vi "Main Loop.vi"(8 "error in (no error)":errorcluster, 10 "Chart Notifier":refnum<notifier>, 11 "Message Queues":T1) -> (0 "error out":errorcluster)   [LabVIEW 2018, in "Feed Module.lvlib" / "Feed Module Engine.lvlib"]
uses:
  Feed Module Engine.lvlib
  Feed Module/Controls/Feed Message Queues.ctl
  support/Message Queue/Message Cluster.ctl
  State Cluster.ctl
  State Enum.ctl
  Feed Module/Controls/Feed Module Settings Cluster.ctl
  Ismatec ISM 831C/Controls/Ismatech ISM831C Settings Cluster.ctl
  Masterflex 7550-30/Controls/Settings Cluster.ctl
  Mettler Toledo/Controls/Settings Cluster.ctl
  Bronkhorst M13 Flow Meter/Settings Cluster.ctl
  PID 2 Parameters Cluster.ctl
  PID Input Enum.ctl
  PID 2 Output Enum.ctl
  Tacmina QI/Tacmina QI DAQ Setting.ctl
  KNF Pump/Settings Cluster plus SIMDOS.ctl
  ASIA Pump/Pump Settings.ctl
  VICI M50 Party Mode/Settings Cluster.ctl
  FLOM Pump/Settings Cluster.ctl
  SSI PR Class/SSI PR or LD Settings Cluster.ctl
  Masterflex 75211/Masterflex 75211 DAQ Setting.ctl
  SSI PR Class/SSI P40 Settings Cluster.ctl
  Ismatec 78001/Ismatec 4083.ctl
  Bronkhorst M14 Flow Meter/Settings Cluster.ctl
  PID 1 Parameters Cluster.ctl
  Feed Module/Controls/Feed Module Display.ctl
  Config Module/Controls/OP Window Display.ctl
  <vilib>/Platform/TimedLoop/XDataNode/timing_clust.ctl
  <vilib>/Platform/TimedLoop/XDataNode/nitl_modes.ctl
  <vilib>/Platform/TimedLoop/XDataNode/wakeup.ctl
  Tag VIs/Tag FGV Operation Enum.ctl
  support/Message Queue/Enqueue Message (Single).vi
  <vilib>/Platform/TimedLoop/XDataNode/XDataNode.xnode
  support/Message Queue/Message Queue.lvlib
  <vilib>/Platform/TimedLoop/XDataNode/XDNodeRunTimeDep.lvlib
  Feed Module/Feed Module.lvlib
  Ismatec ISM 831C/Ismatec ISM 831C.lvlib
  Masterflex 7550-30/Masterflex 7550-30.lvlib
  Bronkhorst M13 Flow Meter/Bronkhorst M13 Flow Meter.lvlib
  Mettler Toledo/Mettler Toledo.lvlib
  Tacmina QI/Tacmina QI.lvlib
  Shared Variables/Dynamic Shared Variables.lvlib
  KNF Pump/KNF SIMDOS.lvlib
  ASIA Pump.lvlib
  VICI M50 Party Mode/VICI M6 M50 Party Mode.lvlib
  FLOM Pump/FLOM Pump.lvlib
  SSI PR Class/SSI PR or LD Pump.lvlib
  support/Support Library.lvlib
  Masterflex 75211/Masterflex 75211.lvlib
  SSI PR Class/SSI P40 Pump.lvlib
  Ismatec 78001/Ismatec 4308.lvlib
  Bronkhorst M14 Flow Meter/Bronkhorst M14 Flow Meter.lvlib
panel:
  out "Period (s)":dbl format="%_4g"
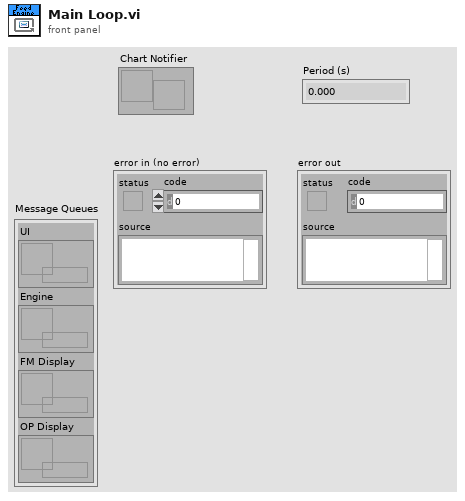
[diagram p1: front panel]
types:
  T1 = typedef "Feed Module.lvlib/Feed Message Queues.ctl" = cluster{"UI":refnum<queue>, "Engine":refnum<queue>, "FM Display":refnum<queue>, "OP Display":refnum<queue>}
  T2 = typedef "XDNodeRunTimeDep.lvlib/timing_clust.ctl" = cluster{"Expected End [f-1]":u64, "Actual End [f-1]":u64, "Finished Late? [f-1]":bool, "Expected End [i-1]":u64, "Actual End [i-1]":u64, "Finished Late? [i-1]":bool, "Expected Start [i]":u64, "Actual Start [i]":u64, "Expected Start [f]":u64, "Actual Start [f]":u64, "Source Name":string, "Structure Name":string, "Period":i64, "Deadline":i64, "Offset":i64, "Start":i64, "Priority":i32, "Timeout":i32, "Mode":T3, "Wakeup Reason":T4, "Error":errorcluster, "Source Type":string, "Secondary Source Type":string, "Global End Time":u64, "Global Start Time":u64, "Frame Duration":u64, "Iteration Duration":u64, "Assigned CPU":i32, "I/O Scan Engine Mode":u32}
  T3 = typedef "XDNodeRunTimeDep.lvlib/nitl_modes.ctl" = enum32{"No Change", "Process missed periods, maintain original phase", "Discard missed periods, maintain original phase", "Process missed periods, ignore original phase", "Discard missed periods, ignore original phase"}
  T4 = typedef "XDNodeRunTimeDep.lvlib/wakeup.ctl" = enum32{"Normal", "Aborted", "Asynchronous wakeup", "Timing source error", "Timed loop error", "Timeout"}
  T5 = cluster{"enable? (F)":bool, "name":string, "alarm on":bool, "priority":u32, "ack type":enum16{"Auto", "User", "None", "Each Occurrence"}, "area":string, "description":string, "log? (T)":bool}
  T6 = typedef "Tag FGV Operation Enum.ctl" = enum16{"Init", "Set Notification Queue", "Create Tag", "Commit", "Write Tag (Numeric)", "Write Tag (Boolean)", "Read All Tags", "Read One Tag", "Delete Tag Category", "Set Alarm Parameters (Numeric)", "Set Alarm Parameters (Boolean)", "Enable All Alarms", "Disable All Alarms", "Delete All Tags", "Read Alarms", "Ack Alarm", "Read Alarm Parameters (Numeric)", "Read Alarm Parameters (Boolean)"}
  T7 = enum32{"u32BitField", "bool", "double", "string", "int8", "uint8", "int16", "uint16", "int32", "uint32", "int64", "uint64", "single", "double waveform", "int16 waveform", "array of boolean", "array of int8", "array of uint8", "array of int16", "array of uint16", "array of int32", "array of uint32", "array of int64", "array of uint64", "array of single", "array of double", "array of double waveform", "array of int16 waveform", "array of string", "variant", "timestamp", "fixed point", "custom"}
  T8 = typedef "Feed Module.lvlib/Feed Module Engine.lvlib/State Enum.ctl" = enum16{"Measuring", "Idle", "Paused"}
  T9 = typedef "Feed Module.lvlib/OP Window Display.ctl" = cluster{"Flow":dbl, "Manual":dbl, "Pump Status":u16, "Smoothed Array":dbl[]}
  T10 = typedef "Feed Module.lvlib/Feed Module Display.ctl" = cluster{"Flow":dbl, "Density":dbl, "FL Temp":dbl, "Scale Value":dbl, "Pump On?":enum16{"Off", "On", "Not Initialized"}, "Cycle Period":dbl, "Input Device":T11, "Output":T12, "Pump's Pressure":dbl, "Pump's Flow ":dbl}
  T11 = typedef "PID Input Enum.ctl" = enum16{"Default", "Bronkhorst M13", "Bronkhorst M14", "Scale Rate of Change"}
  T12 = typedef "PID 2 Output Enum.ctl" = enum16{"Default", "Ismatec ISM 4308", "Ismatec ISM 831C", "Masterflex 7550-30", "VICI", "Tacmina QI", "KNF SIMDOS", "ASIA Type C", "FLOM UI-22-11", "SSI PR/LD", "SSI P40", "Masterflex 75211-70"}
  T13 = typedef "Feed Module.lvlib/Feed Module Engine.lvlib/State Cluster.ctl" = cluster{"State":T8, "Start Time":timestamp, "Configuration":T14, "Current Time":timestamp, "PID 1 Parameters":T30, "First Iteration":bool, "Data":cluster{"Flowmeter Output":dbl, "Density":dbl, "FL Temp":dbl, "Scale Output (g)":dbl, "Scale Rate of Change (g/min)":dbl, "PID 1 Output":dbl, "PID 2 Process Variable":dbl, "PID 2 output":dbl, "Pump Flow":dbl, "Pump Pressure":dbl}, "Process Name":string, "Pump On?":enum16{"Off", "On", "Not Initialized"}, "Input Error":bool, "Output Error":bool, "Log Started":bool, "Current Setpoint":dbl}
  T14 = typedef "Feed Module.lvlib/Feed Module Settings Cluster.ctl" = cluster{"Cycle Period":dbl, "Ismatech":T15, "Masterflex":T16, "Mettler":T17, "Bronkhorst M13 Flow Meter":T18, "PID 2 Parameters":T19, "Manual Entry":dbl, "Auto?":bool, "output range":cluster{"output high":dbl, "output low":dbl}, "Tacmina Settings":T20, "KNF SIMDOS Settings":T21, "ASIA Pump C":T22, "VICI Settings":T23, "FLOM Settings":T24, "SSI PR/LD Settings":T25, "Masterflex 75211 Settings":T26, "SSI P40 Settings":T27, "Ismatech 3 Channel Settings":T28, "Bronkhorst M14 Settings":T29}
  T15 = typedef "Ismatec ISM 831C.lvlib/Ismatech ISM831C Settings Cluster.ctl" = cluster{"VISA resource name":refnum<visa-resource-name>, "Simulated?":bool, "Pump Number":dbl, "Reverse?":bool}
  T16 = typedef "Masterflex 7550-30.lvlib/Settings Cluster.ctl" = cluster{"VISA resource name":refnum<visa-resource-name>, "Simulated?":bool, "Pump Number":dbl, "Reverse?":bool}
  T17 = typedef "Mettler Toledo.lvlib/Settings Cluster.ctl" = cluster{"VISA resource name":refnum<visa-resource-name>, "Simulated?":bool}
  T18 = typedef "Bronkhorst M13 Flow Meter.lvlib/Settings Cluster.ctl" = cluster{"VISA resource name":refnum<visa-resource-name>, "Simulated?":bool, "Smoothing Steps":i32}
  T19 = typedef "PID 2 Parameters Cluster.ctl" = cluster{"Input Device":T11, "Output Device":T12, "Setpoint":dbl, "PID gains":cluster{"proportional gain (Kc)":dbl, "integral time (Ti, min)":dbl, "derivative time (Td, min)":dbl}}
  T20 = typedef "Tacmina QI.lvlib/Tacmina QI DAQ Setting.ctl" = cluster{"Analog DAQ Task":refnum<k21>, "Digital DAQ Task":refnum<k21>}
  T21 = typedef "KNF SIMDOS.lvlib/Settings Cluster plus SIMDOS.ctl" = cluster{"VISA resource name":refnum<visa-resource-name>, "Simulated?":bool}
  T22 = typedef "ASIA Pump.lvlib/Pump Settings.ctl" = cluster{"ASIA Pump #":i32, "channel":i32, "Simulated":bool}
  T23 = typedef "VICI M6 M50 Party Mode.lvlib/Settings Cluster.ctl" = cluster{"VISA resource name":refnum<visa-resource-name>, "Simulated?":bool, "Pump Letter":string, "Reverse?":bool}
  T24 = typedef "FLOM Pump.lvlib/Settings Cluster.ctl" = cluster{"VISA resource name":refnum<visa-resource-name>, "Simulated?":bool, "Pump Number":dbl}
  T25 = typedef "SSI PR or LD Pump.lvlib/SSI PR or LD Settings Cluster.ctl" = cluster{"VISA resource name":refnum<visa-resource-name>, "Simulated?":bool}
  T26 = typedef "Masterflex 75211.lvlib/Masterflex 75211 DAQ Setting.ctl" = cluster{"Analog DAQ Task":refnum<k21>, "Digital DAQ Task":refnum<k21>}
  T27 = typedef "SSI P40 Pump.lvlib/SSI P40 Settings Cluster.ctl" = cluster{"VISA resource name":refnum<visa-resource-name>, "Simulated?":bool}
  T28 = typedef "Ismatec 4308.lvlib/Ismatec 4083.ctl" = cluster{"VISA resource name":refnum<visa-resource-name>, "Pump Number":i16, "Channel Number":i16, "Simulated?":bool, "Reverse?":bool}
  T29 = typedef "Bronkhorst M14 Flow Meter.lvlib/Settings Cluster.ctl" = cluster{"VISA resource name":refnum<visa-resource-name>, "Simulated?":bool, "Smoothing Steps":i32}
  T30 = typedef "PID 1 Parameters Cluster.ctl" = cluster{"Setpoint":dbl, "PID gains":cluster{"proportional gain (Kc)":dbl, "integral time (Ti, min)":dbl, "derivative time (Td, min)":dbl}}
  T31 = cluster{"Flowmeter Output":dbl, "Density":dbl, "FL Temp":dbl, "Scale Output (g)":dbl, "Scale Rate of Change (g/min)":dbl, "PID 1 Output":dbl, "PID 2 Process Variable":dbl, "PID 2 output":dbl, "Pump Flow":dbl, "Pump Pressure":dbl}
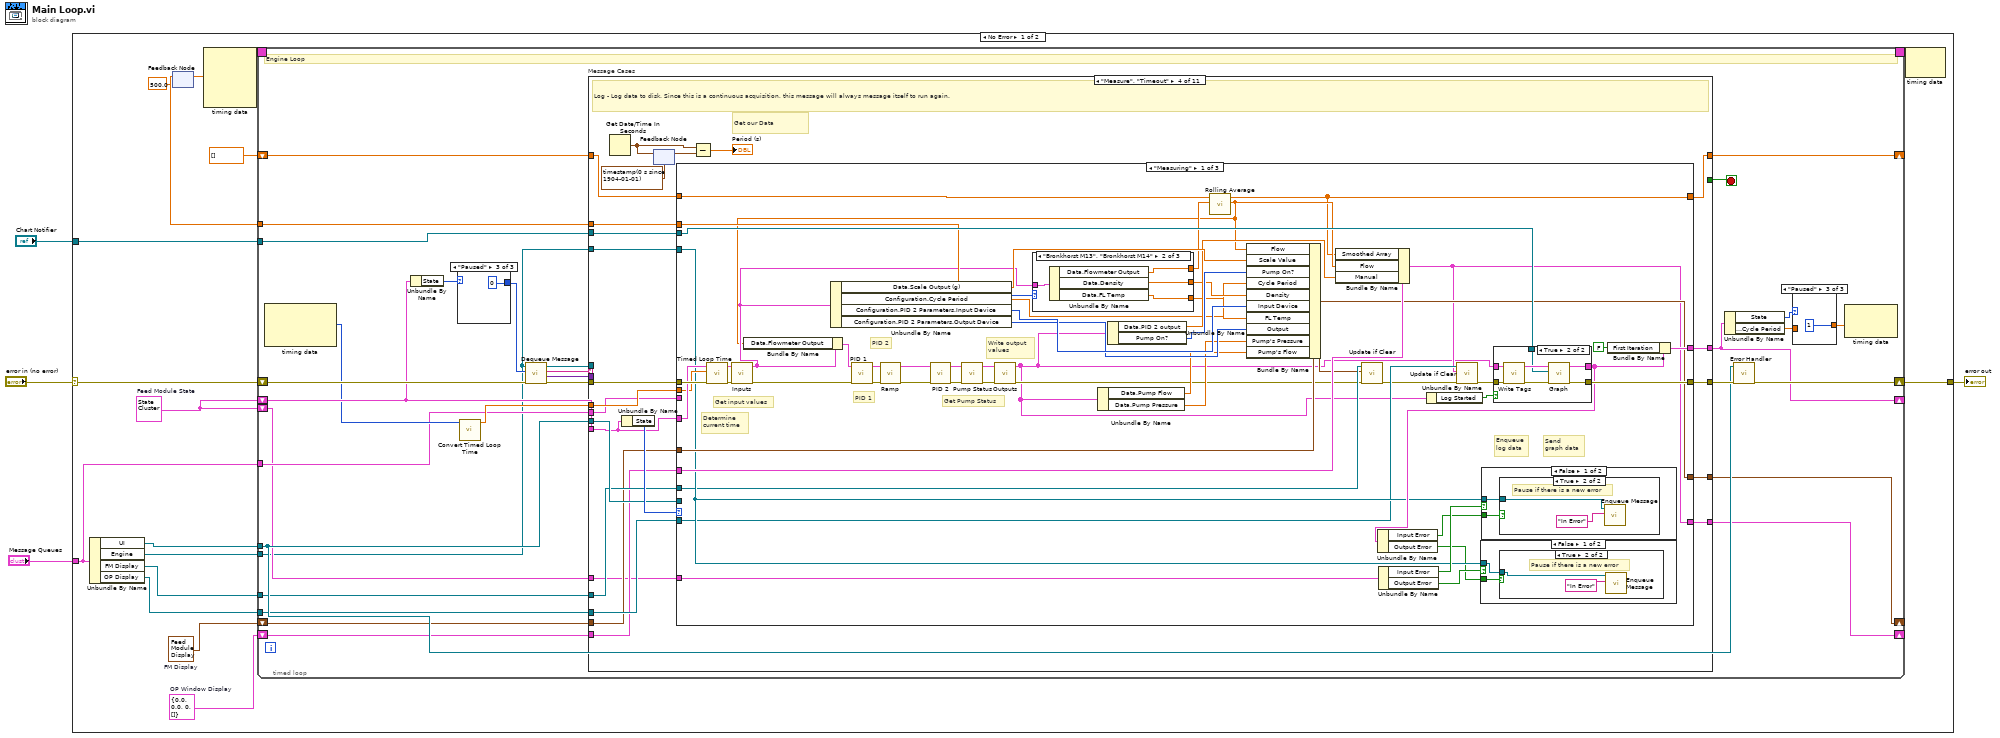
[diagram p0: block diagram]
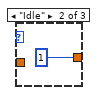
[diagram p3: hidden frame]
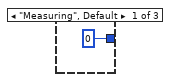
[diagram p4: hidden frame]
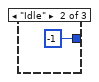
[diagram p5: hidden frame]
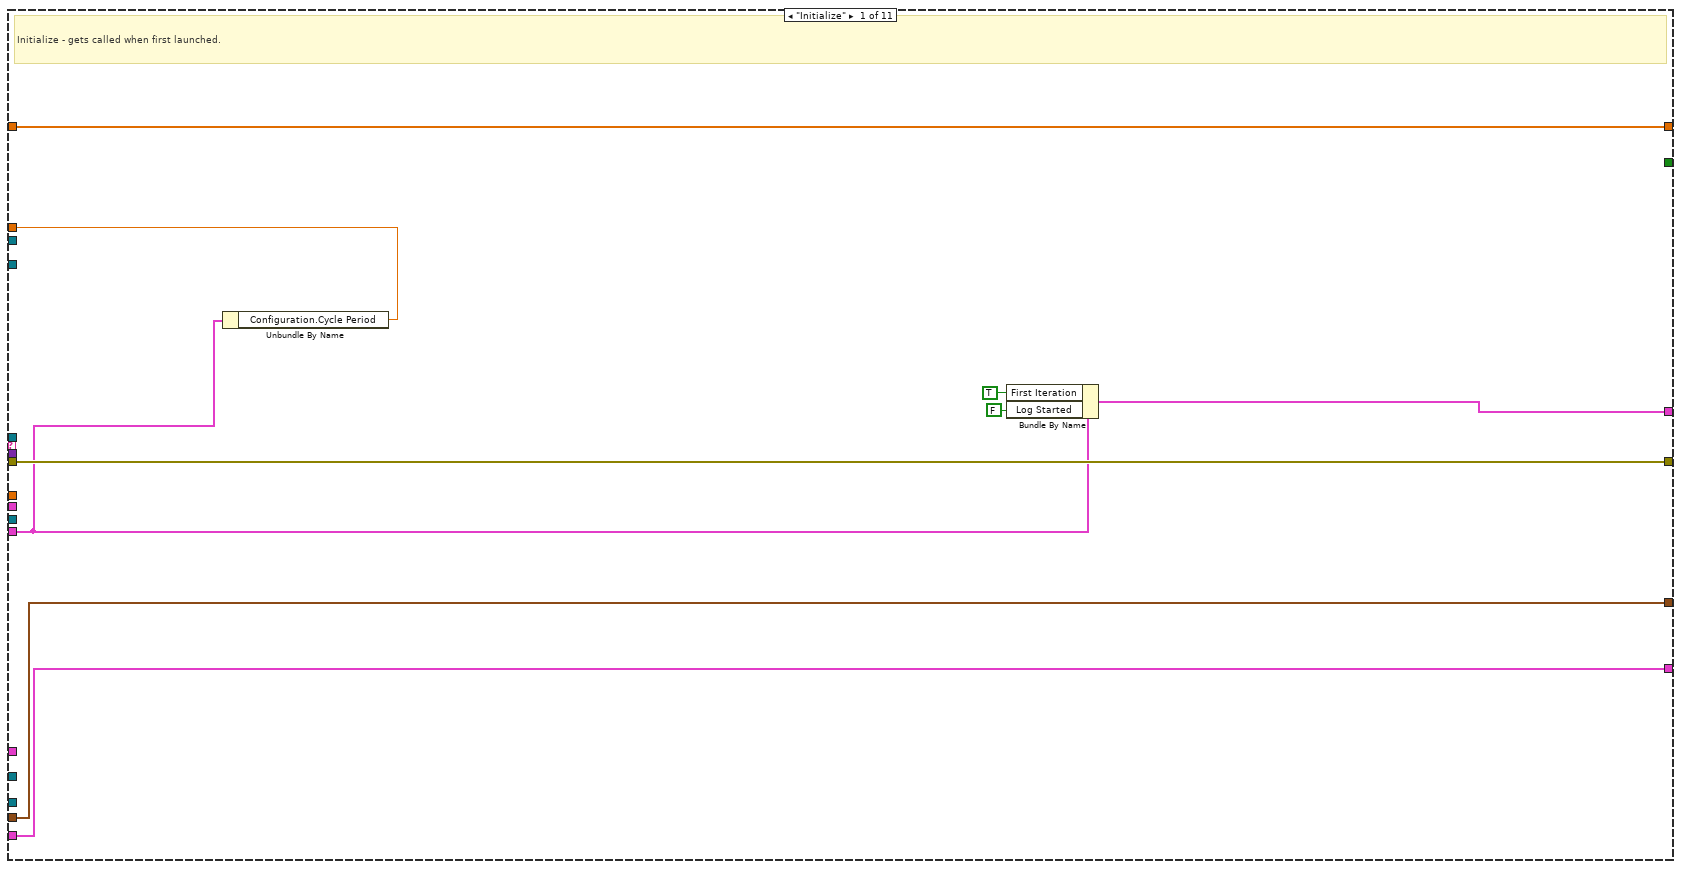
[diagram p6: hidden frame]
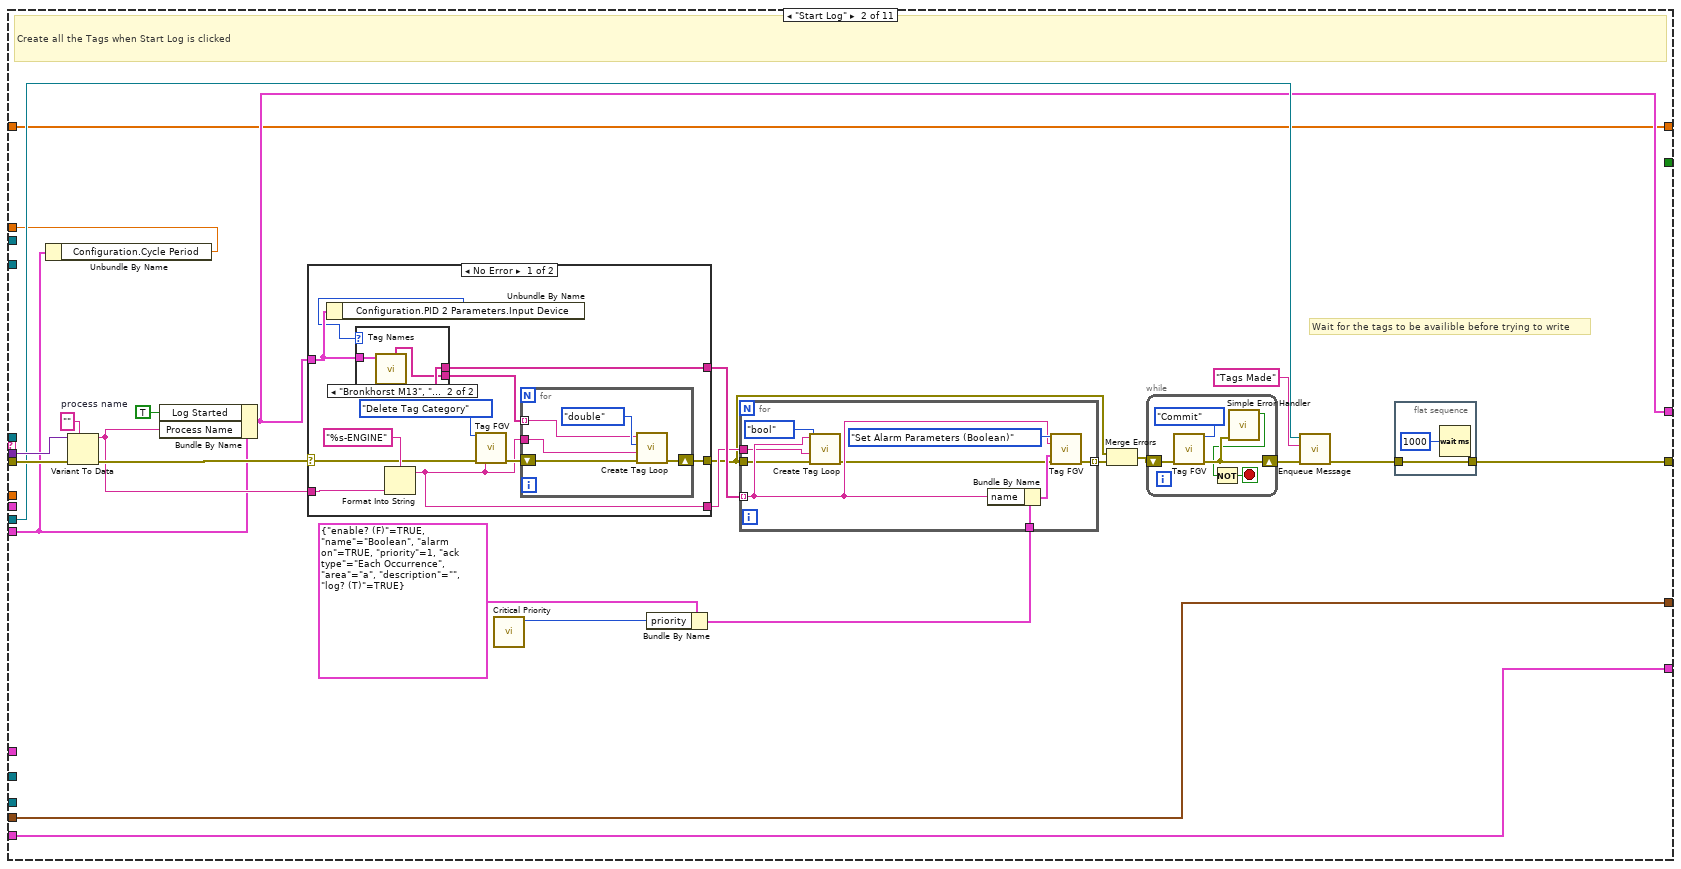
[diagram p7: hidden frame]
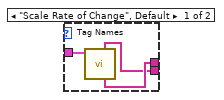
[diagram p8: hidden frame]
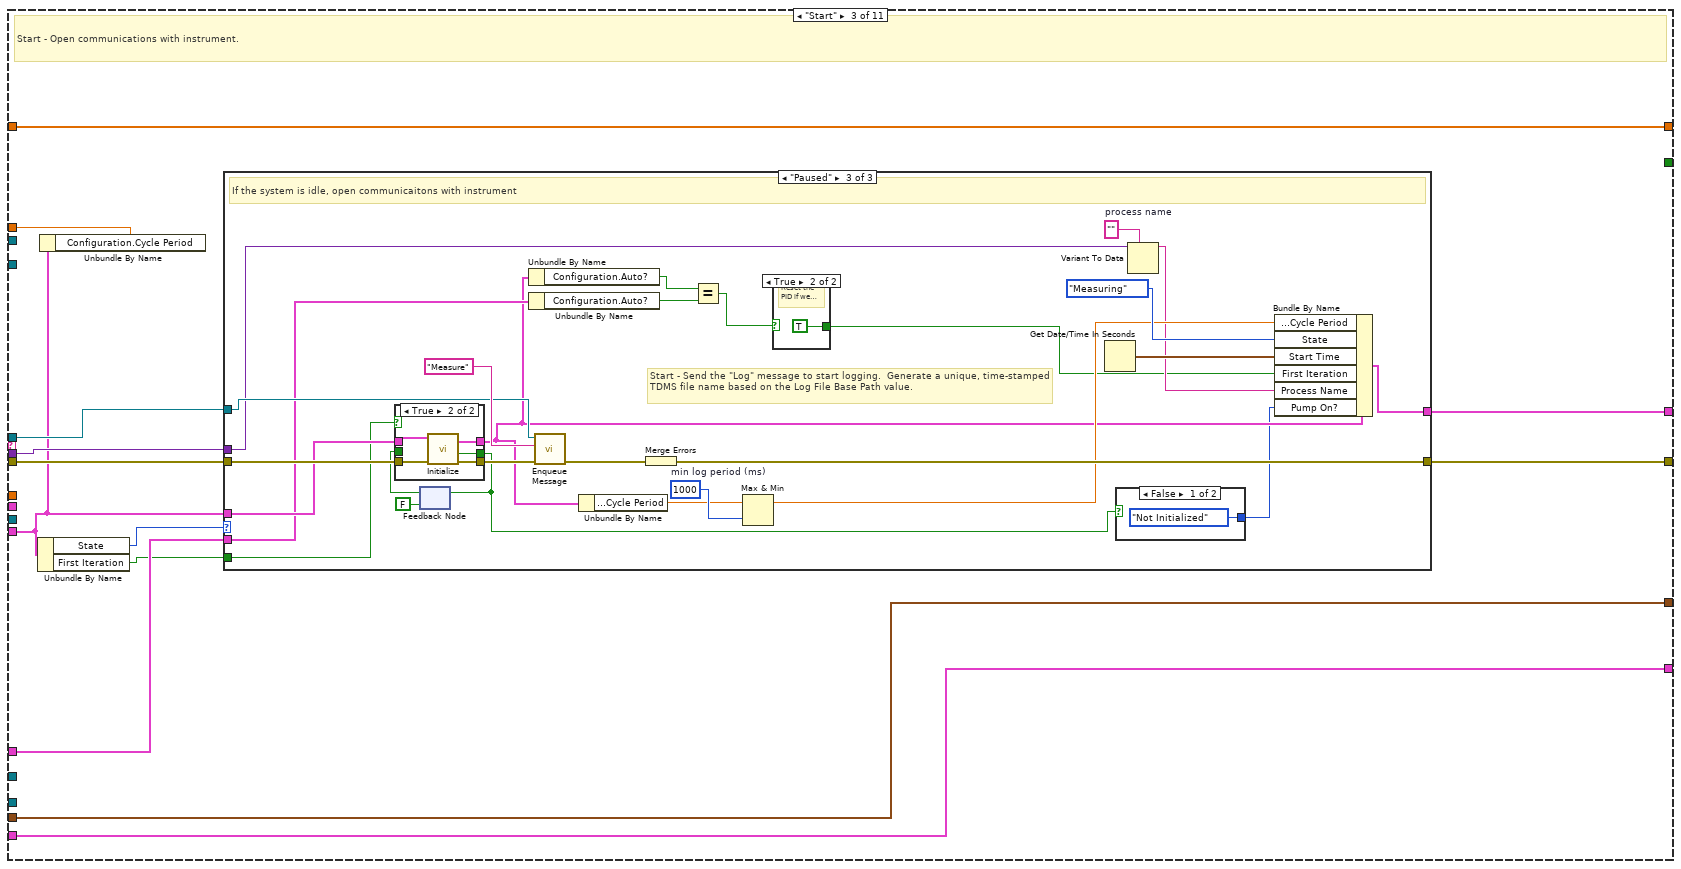
[diagram p10: hidden frame]
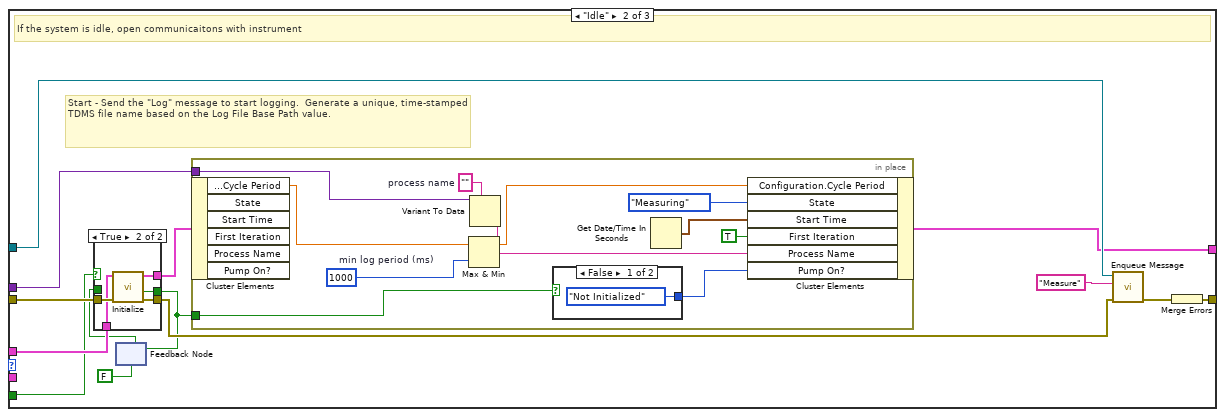
[diagram p12: hidden frame]
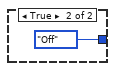
[diagram p13: hidden frame]
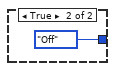
[diagram p16: hidden frame]
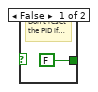
[diagram p17: hidden frame]
diagram:
  n1 = case shown="No Error" "error in (no error)" {
    selector: "error in (no error)" -> [w20 w593]
    tunnel: "Message Queues" -> [w16 _]
    tunnel: [w21 w593] -> w3
    tunnel: "Chart Notifier" -> [w14 _]
    frame No Error {
      w11 = T9 {"Flow"=0.0, "Manual"=0.0, "Pump Status"=0, "Smoothed Array"=[]}  # OP Window Display
      w9 = T10 {"Flow"=0.0, "Density"=0.0, "FL Temp"=0.0, "Scale Value"=0.0, "Pump On?"=enum."Off", "Cycle Period"=500.0, "Input Device"=enum."Bronkhorst M13", "Output"=enum."Default", "Pump's Pressure"=0.0, "Pump's Flow "=0.0}  # FM Display
      w12 = T13 {"State"=enum."Idle", "Start Time"=timestamp(0 s since 1904-01-01), "Configuration"={"Cycle Period"=0.0, "Ismatech"={"VISA resource name"="", "Simulated?"=FALSE, "Pump Number"=1.0, "Reverse?"=FALSE}, "Masterflex"={"VISA resource name"="", "Simulated?"=FALSE, "Pump Number"=1.0, "Reverse?"=FALSE}, "Mettler"={"VISA resource name"="", "Simulated?"=FALSE}, "Bronkhorst M13 Flow Meter"={"VISA resource name"="", "Simulated?"=FALSE, "Smoothing Steps"=1}, "PID 2 Parameters"={"Input Device"=enum."Bronkhorst M13", "Output Device"=enum."Ismatec ISM 831C", "Setpoint"=0.0, "PID gains"={"proportional gain (Kc)"=1.0, "integral time (Ti, min)"=0.01, "derivative time (Td, min)"=0.0}}, "Manual Entry"=0.0, "Auto?"=TRUE, "output range"={"output high"=100.0, "output low"=0.0}, "Tacmina Settings"={"Analog DAQ Task"="", "Digital DAQ Task"=""}, "KNF SIMDOS Settings"={"VISA resource name"="", "Simulated?"=TRUE}, "ASIA Pump C"={"ASIA Pump #"=0, "channel"=0, "Simulated"=FALSE}, "VICI Settings"={"VISA resource name"="", "Simulated?"=FALSE, "Pump Letter"="", "Reverse?"=FALSE}, "FLOM Settings"={"VISA resource name"="", "Simulated?"=TRUE, "Pump Number"=0.0}, "SSI PR/LD Settings"={"VISA resource name"="", "Simulated?"=FALSE}, "Masterflex 75211 Settings"={"Analog DAQ Task"="", "Digital DAQ Task"=""}, "SSI P40 Settings"={"VISA resource name"="", "Simulated?"=TRUE}, "Ismatech 3 Channel Settings"={"VISA resource name"="", "Pump Number"=1, "Channel Number"=0, "Simulated?"=TRUE, "Reverse?"=FALSE}, "Bronkhorst M14 Settings"={"VISA resource name"="", "Simulated?"=FALSE, "Smoothing Steps"=1}}, "Current Time"=timestamp(0 s since 1904-01-01), "PID 1 Parameters"={"Setpoint"=0.0, "PID gains"={"proportional gain (Kc)"=1.0, "integral time (Ti, min)"=0.01, "derivative time (Td, min)"=0.0}}, "First Iteration"=FALSE, "Data"={"Flowmeter Output"=0.0, "Density"=0.0, "FL Temp"=0.0, "Scale Output (g)"=0.0, "Scale Rate of Change (g/min)"=0.0, "PID 1 Output"=0.0, "PID 2 Process Variable"=0.0, "PID 2 output"=0.0, "Pump Flow"=0.0, "Pump Pressure"=0.0}, "Process Name"="", "Pump On?"=enum."Off", "Input Error"=FALSE, "Output Error"=FALSE, "Log Started"=FALSE, "Current Setpoint"=0.0}  # Feed Module State
      n2 = Unbundle By Name(w16) -> ("UI"=w19:refnum<queue>, "Engine"=w15:refnum<queue>, "FM Display"=w13:refnum<queue>, "OP Display"=w10:refnum<queue>)
      n3 = feedback #1(500.0 ("Cycle Period")) -> (w7:dbl)
      n4 = node-c288(w7) -> (w18:T2)  [unwired: 3 in]
      n5 = timed-loop {
        tunnel: w15 -> [w27]
        shift-right: [w41] -> _
        shift-left: w12 -> [w44]
        shift-right: [w46] -> w21
        shift-left: w20 -> [w52]
        tunnel: w19 -> [w45]
        timing: w18 -> [_]
        timing-out: [_] -> w17
        tunnel: w16 -> [w35]
        tunnel: w14 -> [w34]
        tunnel: w13 -> [w33]
        tunnel: w10 -> [w32]
        shift-right: [w31] -> _
        shift-left: w9 -> [w25]
        shift-right: [w30] -> _
        shift-left: w11 -> [w26]
        shift-left: w12 -> [w29]
        tunnel: [w24] -> w8
        shift-right: [w22] -> _
        shift-left: dbl[] [] -> [w23]
        stop <- w28 stop-if-true
        # "Engine Loop"
        n6 = node-c288() -> (w37:i64)  [unwired: 1 in, 2 out]
        n7 = Unbundle By Name(w44) -> ("State"=w43:T8)
        n8 = case shown="\"Paused\"" w43 {
          tunnel: [0 ("timeout in ms (-1)") -1 ("timeout in ms (-1)") 0 ("timeout in ms (-1)")] -> w42
          frame "Measuring", Default {
          }
          frame "Idle" {
          }
          frame "Paused" {
          }
        }
        n9 = call "Convert Timed Loop Time.vi"("Actual Start [i]"=w37) -> ("ET since start (s)"=w36:dbl)  [unwired: 10 in]
        n10 = call "Dequeue Message.vi"("error in (no error)"=w52, "timeout in ms (-1)"=w42, "Message Queue"=w27) -> ("error out"=w51:errorcluster, "Message Data"=w49:variant, "Message"=w50:string, "dup Message Queue"=w48:refnum<queue>)  [unwired: 5 in]
        n11 = case "Message Cases" shown="\"Measure\", \"Timeout\"" w50 {
          selector: w50 -> [_ _ _ _ _ _ _ _ _ _ w579]
          tunnel: w48 -> [_ _ w148 _ w431 _ _ w516 _ w541 _]
          tunnel: w51 -> [w72 w93 w147 w246 w427 w455 w504 w519 w529 w563 _]
          tunnel: [w72 w75 w149 w247 w418 w445 w498 w521 w528 w559 w580] -> w47
          tunnel: w44 -> [w66 w79 w139 w244 w426 w452 w500 w511 w525 w558 w586]
          tunnel: [w69 w81 w146 w245 w424 w449 w496 w511 w525 w560 w586] -> w41
          tunnel: [_ _ _ _ _ _ _ TRUE _ _ _] -> w28
          tunnel: w49 -> [_ w94 w144 _ _ _ w505 _ _ _ _]
          tunnel: w45 -> [_ w82 _ w248 w430 w459 _ w520 _ _ _]
          tunnel: w36 -> [_ _ _ w243 _ _ _ _ _ _ _]
          tunnel: w35 -> [_ _ _ w242 _ _ _ _ _ _ _]
          tunnel: w34 -> [_ _ _ w238 _ _ _ _ _ _ _]
          tunnel: w33 -> [_ _ _ w237 w423 w450 _ _ _ w540 _]
          tunnel: w32 -> [_ _ _ w236 w421 w447 _ _ _ w539 _]
          tunnel: w25 -> [w70 w97 w143 w235 w428 w457 w502 w513 w527 w556 w588]
          tunnel: [w70 w97 w143 w234 w428 w457 w502 w513 w527 w538 w588] -> w31
          tunnel: w26 -> [w71 w96 w142 w233 w420 w446 w501 w512 w526 w555 w587]
          tunnel: [w71 w96 w142 w232 w420 w446 w501 w512 w526 w537 w587] -> w30
          tunnel: w29 -> [_ _ w141 w231 _ _ _ _ _ _ _]
          tunnel: w27 -> [_ _ _ w230 _ _ _ _ _ _ _]
          tunnel: [w67 w80 w138 w229 w425 w451 w497 w510 w524 w557 w585] -> w24
          tunnel: w23 -> [w64 w73 w137 w227 w417 w443 _ w509 w523 w533 w578]
          tunnel: [w64 w73 w137 w226 w417 w443 w490 w509 w523 w532 w578] -> w22
          frame "Initialize" {
            # "Initialize - gets called when first launched."
            n12 = Unbundle By Name(w66) -> ("Configuration.Cycle Period"=w67:dbl)
            n13 = Bundle By Name(cluster=w66, "First Iteration"=TRUE, "Log Started"=FALSE) -> (w69:T13)
          }
          frame "Start Log" {
            w95 = ""  # process name
            # "Wait for the tags to be availible before trying to write"
            # "Create all the Tags when Start Log is clicked"
            n14 = Unbundle By Name(w79) -> ("Configuration.Cycle Period"=w80:dbl)
            n15 = Variant To Data(error in=w93, type=w95, Variant=w94) -> (data=w91:string, error out=w92:errorcluster)
            n16 = Bundle By Name(cluster=w79, "Log Started"=TRUE, "Process Name"=w91) -> (w81:T13)
            n17 = case shown="No Error" w92 {
              selector: w92 -> [w121 w136]
              tunnel: [w124 w136] -> w74
              tunnel: w91 -> [w119 _]
              tunnel: [w118 _] -> w87
              tunnel: [w117 _] -> w85
              tunnel: w81 -> [w115 _]
              frame No Error {
                n18 = Unbundle By Name(w115) -> ("Configuration.PID 2 Parameters.Input Device"=w114:T11)
                n19 = case shown="\"Bronkhorst M13\", \"Bronkhorst M14\"" w114 {
                  tunnel: [w126 w130] -> w118
                  tunnel: [w125 w128] -> w116
                  tunnel: w115 -> [w127 w129]
                  frame "Scale Rate of Change", Default {
                    n20 = call "Tag Names.vi"("State in"=w127) -> ("All Boolean Tags"=w126:string[], "All  Numeric Tags"=w125:string[])  [unwired: 6 in, 3 out]
                  }
                  frame "Bronkhorst M13", "Bronkhorst M14" {
                    n21 = call "Tag Names.vi"("State in"=w129) -> ("All Boolean Tags"=w130:string[], "All  Numeric Tags"=w128:string[])  [unwired: 6 in, 3 out]
                  }
                }
                n22 = Format Into String(format string="%s-ENGINE", w119) -> (resulting string=w117:string)  [unwired: 2 in, 1 out]
                n23 = call "Tag FGV.vi"("Operation"=Tag_FGV_Operation_Enum."Delete Tag Category", "error in (no error)"=w121, "Tag Category"=w117) -> ("error out"=w120:errorcluster)  [unwired: 5 in, 7 out]
                n24 = for {
                  tunnel: w116 -> [w132] mode=indexing
                  shift-right: [w131] -> w124
                  shift-left: w120 -> [w134]
                  tunnel: w117 -> [w133]
                  n25 = call "Create Tag Loop.vi"("error in (no error)"=w134, "Tag Category"=w133, "data type"=T7."double", "Tag Name"=w132) -> ("error out"=w131:errorcluster)  [unwired: 7 in]
                }
              }
              frame Error {
              }
            }
            n26 = call "Critical Priority.vi"() -> ("critical priority"=w89:i32)  [unwired: 11 in]
            n27 = Bundle By Name(cluster=T5 {"enable? (F)"=TRUE, "name"="Boolean", "alarm on"=TRUE, "priority"=1, "ack type"=enum."Each Occurrence", "area"="a", "description"="", "log? (T)"=TRUE} ("Boolean alarm settings"), "priority"=w89) -> (w88:T5)
            n28 = for {
              tunnel: w88 -> [w113]
              tunnel: [w112] -> w86 mode=indexing
              tunnel: w87 -> [w108] mode=indexing
              tunnel: w74 -> [w106]
              tunnel: w85 -> [w107]
              n29 = call "Create Tag Loop.vi"("error in (no error)"=w106, "Tag Category"=w107, "data type"=T7."bool", "Tag Name"=w108) -> ("error out"=w105:errorcluster)  [unwired: 7 in]
              n30 = Bundle By Name(cluster=w113, "name"=w108) -> (w111:T5)
              n31 = call "Tag FGV.vi"("Operation"=Tag_FGV_Operation_Enum."Set Alarm Parameters (Boolean)", "Tag Name"=w108, "Data"=w111, "error in (no error)"=w105) -> ("error out"=w112:errorcluster)  [unwired: 4 in, 7 out]
            }
            n32 = Merge Errors(w74, w86) -> (w78:errorcluster)
            n33 = while {
              shift-right: [w102] -> w77
              shift-left: w78 -> [w103]
              stop <- w100 stop-if-true
              n34 = call "Tag FGV.vi"("Operation"=Tag_FGV_Operation_Enum."Commit", "error in (no error)"=w103) -> ("error out"=w102:errorcluster)  [unwired: 6 in, 7 out]
              n35 = call <vilib>:"Simple Error Handler.vi"("error in (no error)"=w102) -> ("error?"=w101:bool)  [unwired: 4 in, 4 out]
              n36 = Not(x=w101) -> (.not. x?=w100:bool)
            }
            n37 = call-poly "Enqueue Message.vi"("error in (no error)"=w77, "Message"="Tags Made", "Message Queue"=w82) -> ("error out"=w76:errorcluster)  [unwired: 7 in, 1 out]
            n38 = flat-sequence {
              tunnel: w76 -> [w98]
              tunnel: [w98] -> w75
              frame #0 {
                n39 = Wait (ms)(milliseconds to wait=u32 1000) -> ()  [unwired: 1 out]
              }
            }
          }
          frame "Start" {
            # "Start - Open communications with instrument."
            n40 = Unbundle By Name(w139) -> ("State"=w145:T8, "First Iteration"=w140:bool)
            n41 = Unbundle By Name(w139) -> ("Configuration.Cycle Period"=w138:dbl)
            n42 = case shown="\"Paused\"" w145 {
              tunnel: [w150 w165 w213] -> w149
              tunnel: w148 -> [_ w162 w204]
              tunnel: w147 -> [w150 w161 w202]
              tunnel: w139 -> [w151 w160 w201]
              tunnel: [w151 w153 w211] -> w146
              tunnel: w144 -> [_ w159 w199]
              tunnel: w141 -> [_ _ w195]
              tunnel: w140 -> [_ w155 w190]
              frame "Measuring", Default {
                # "The system is already running. Ignore the \"Start\" message."
              }
              frame "Idle" {
                # "Start - Send the \"Log\" message to start logging.  Generate a unique, time-stamped TDMS file name based on the Log File Base Path value."
                # "If the system is idle, open communicaitons with instrument"
                n43 = feedback #2(FALSE ("Pump Initialized")) -> (w157:bool)
                n44 = case shown="True" w155 {
                  tunnel: w161 -> [w180 w186]
                  tunnel: w160 -> [w181 w185]
                  tunnel: [w181 w184] -> w154
                  tunnel: [w180 w183] -> w158
                  tunnel: [w179 w182] -> w156
                  tunnel: w157 -> [w179 _]
                  frame False {
                  }
                  frame True {
                    n45 = call "Initialize.vi"("error in (no error)"=w186, "State in"=w185) -> ("error out"=w183:errorcluster, "Pump Initialized"=w182:bool, "State out"=w184:T13)  [unwired: 7 in]
                  }
                }
                n46 = feedback-in #2(w156) -> ()
                n47 = in-place {
                  in-place-border: w159 -> [w174]
                  in-place-border: w156 -> [w173]
                  w175 = ""  # process name
                  w176 = 1000  # min log period (ms)
                  n48 = in-place-cluster #3(w154) -> ("Configuration.Cycle Period"=w172:dbl)  [unwired: 5 out]
                  n49 = Max & Min(x=w172, y=w176) -> (max(x,y)=w171:dbl)  [unwired: 1 out]
                  n50 = Variant To Data(type=w175, Variant=w174) -> (data=w167:string)  [unwired: 1 in, 1 out]
                  n51 = case shown="False" w173 {
                    tunnel: [enum16{"Off", "On", "Not Initialized"}."Not Initialized" ("Pump On?") enum16{"Off", "On", "Not Initialized"}."Off" ("Pump On?")] -> w166
                    frame False {
                    }
                    frame True {
                    }
                  }
                  n52 = Get Date/Time In Seconds() -> (seconds since 1Jan1904=w169:timestamp)
                  n53 = in-place-cluster #3("Configuration.Cycle Period"=w171, "State"=State_Enum."Measuring", "Start Time"=w169, "First Iteration"=TRUE, "Process Name"=w167, "Pump On?"=w166) -> (w153:T13)
                }
                n54 = call-poly "Enqueue Message.vi"("error in (no error)"=w158, "Message"="Measure", "Message Queue"=w162) -> ("error out"=w163:errorcluster)  [unwired: 7 in, 1 out]
                n55 = Merge Errors(w163) -> (w165:errorcluster)
              }
              frame "Paused" {
                w200 = ""  # process name
                w208 = 1000  # min log period (ms)
                # "Start - Send the \"Log\" message to start logging.  Generate a unique, time-stamped TDMS file name based on the Log File Base Path value."
                # "If the system is idle, open communicaitons with instrument"
                n56 = feedback #4(FALSE ("Pump Initialized")) -> (w189:bool)
                n57 = case shown="True" w190 {
                  tunnel: [w216 w221] -> w203
                  tunnel: w202 -> [w216 w220]
                  tunnel: w201 -> [w215 w219]
                  tunnel: [w215 w218] -> w192
                  tunnel: [w214 w217] -> w188
                  tunnel: w189 -> [w214 _]
                  frame False {
                  }
                  frame True {
                    n58 = call "Initialize.vi"("error in (no error)"=w220, "State in"=w219) -> ("error out"=w221:errorcluster, "Pump Initialized"=w217:bool, "State out"=w218:T13)  [unwired: 7 in]
                  }
                }
                n59 = feedback-in #4(w188) -> ()
                n60 = Unbundle By Name(w192) -> ("Configuration.Auto?"=w196:bool)
                n61 = Unbundle By Name(w195) -> ("Configuration.Auto?"=w194:bool)
                n62 = call-poly "Enqueue Message.vi"("error in (no error)"=w203, "Message"="Measure", "Message Queue"=w204) -> ("error out"=w209:errorcluster)  [unwired: 7 in, 1 out]
                n63 = Unbundle By Name(w192) -> ("Configuration.Cycle Period"=w207:dbl)
                n64 = Merge Errors(w209) -> (w213:errorcluster)
                n65 = Equal?(x=w196, y=w194) -> (x = y?=w197:bool)
                n66 = Max & Min(x=w207, y=w208) -> (max(x,y)=w206:dbl)  [unwired: 1 out]
                n67 = case shown="True" w197 {
                  tunnel: [FALSE ("First Iteration") TRUE ("First Iteration")] -> w193
                  frame False {
                    # "Don't reset the PID if we are switching Auto?"
                  }
                  frame True {
                    # "Reset the PID if we start from paused"
                  }
                }
                n68 = Get Date/Time In Seconds() -> (seconds since 1Jan1904=w205:timestamp)
                n69 = case shown="False" w188 {
                  tunnel: [enum16{"Off", "On", "Not Initialized"}."Not Initialized" ("Pump On?") enum16{"Off", "On", "Not Initialized"}."Off" ("Pump On?")] -> w191
                  frame False {
                  }
                  frame True {
                  }
                }
                n70 = Variant To Data(type=w200, Variant=w199) -> (data=w198:string)  [unwired: 1 in, 1 out]
                n71 = Bundle By Name(cluster=w192, "Configuration.Cycle Period"=w206, "State"=State_Enum."Measuring", "Start Time"=w205, "First Iteration"=w193, "Process Name"=w198, "Pump On?"=w191) -> (w211:T13)
              }
            }
          }
          frame "Measure", "Timeout" {
            # "Get our Data"
            # "Log - Log data to disk. Since this is a continuous acquisition, this message will always message itself to run again."
            n72 = Get Date/Time In Seconds() -> (seconds since 1Jan1904=w240:timestamp)
            n73 = Unbundle By Name(w244) -> ("State"=w249:T8)
            n74 = feedback-in #5(w240) -> ()
            n75 = feedback #5(timestamp(0 s since 1904-01-01) ("seconds since 1Jan1904")) -> (w241:timestamp)
            n76 = case shown="\"Measuring\"" w249 {
              tunnel: w246 -> [w299 w335 w366]
              tunnel: w244 -> [w297 w339 w367]
              tunnel: w248 -> [_ _ _]
              tunnel: [w301 w331 w344] -> w247
              tunnel: [w294 w339 w361] -> w245
              tunnel: w243 -> [w295 _ w383]
              tunnel: w242 -> [_ _ _]
              tunnel: w238 -> [w292 _ w384]
              tunnel: w237 -> [w263 w337 w350]
              tunnel: w236 -> [w260 w334 w347]
              tunnel: w235 -> [w287 w336 w381]
              tunnel: [w262 w336 w349] -> w234
              tunnel: w233 -> [w286 w333 w382]
              tunnel: [w259 w333 w346] -> w232
              tunnel: w231 -> [w268 _ w376]
              tunnel: w230 -> [w279 _ w373]
              tunnel: [w267 w338 w353] -> w229
              tunnel: w227 -> [w256 w330 w343]
              tunnel: [w250 w330 w342] -> w226
              frame "Measuring" {
                # "Get Pump Status"
                # "Send\ngraph data"
                # "Enqueue\nlog data"
                # "PID 2"
                # "PID 1"
                # "Determine\ncurrent time"
                # "Write output\nvalues"
                # "Get input values"
                n77 = call "Timed Loop Time.vi"("error in (no error)"=w299, "ET since start (s)"=w295, "State in"=w297) -> ("error out"=w300:errorcluster, "State out"=w298:T13)  [unwired: 7 in]
                n78 = call "Inputs.vi"("error in (no error)"=w300, "State in"=w298) -> ("error out"=w296:errorcluster, "State out"=w254:T13)  [unwired: 8 in]
                n79 = Unbundle By Name(w254) -> ("Data.Scale Output (g)"=w285:dbl, "Configuration.Cycle Period"=w267:dbl, "Configuration.PID 2 Parameters.Input Device"=w276:T11, "Configuration.PID 2 Parameters.Output Device"=w266:T12)
                n80 = case shown="\"Bronkhorst M13\", \"Bronkhorst M14\"" w276 {
                  tunnel: w254 -> [_ w325 w329]
                  tunnel: [0.0 ("Scale Rate of Change (g/min)") w324 w328] -> w255
                  tunnel: [0.0 ("Density") w323 nan ("Density")] -> w275
                  tunnel: [0.0 ("Density") w322 nan ("Density")] -> w274
                  frame "Default", Default {
                  }
                  frame "Bronkhorst M13", "Bronkhorst M14" {
                    n81 = Unbundle By Name(w325) -> ("Data.Flowmeter Output"=w324:dbl, "Data.Density"=w323:dbl, "Data.FL Temp"=w322:dbl)
                  }
                  frame "Scale Rate of Change" {
                    n82 = Unbundle By Name(w329) -> ("Data.Scale Rate of Change (g/min)"=w328:dbl)
                  }
                }
                n83 = call "Rolling Average.vi"("New Value"=w255, "Old Array"=w256) -> ("Calculated Value"=w251:dbl, "New Array"=w250:dbl[])  [unwired: 8 in]
                n84 = Bundle By Name(cluster=w254, "Data.Flowmeter Output"=w251) -> (w253:T13)
                n85 = call "PID 1.vi"("error in (no error)"=w296, "State in"=w253) -> ("error out"=w271:errorcluster, "State out"=w272:T13)  [unwired: 8 in]
                n86 = call "Ramp.vi"("error in (no error)"=w271, "State in"=w272) -> ("error out"=w270:errorcluster, "State Out"=w269:T13)  [unwired: 8 in]
                n87 = call "PID 2.vi"("error in (no error)"=w270, "State in"=w269) -> ("error out"=w289:errorcluster, "State out"=w291:T13)  [unwired: 8 in]
                n88 = call "Pump Status.vi"("error in (no error)"=w289, "State in"=w291) -> ("error out"=w288:errorcluster, "State out"=w290:T13)  [unwired: 8 in]
                n89 = call "Outputs.vi"("error in (no error)"=w288, "State in"=w290) -> ("error out"=w261:errorcluster, "State out"=w252:T13)  [unwired: 8 in]
                n90 = Unbundle By Name(w252) -> ("Data.Pump Flow"=w265:dbl, "Data.Pump Pressure"=w264:dbl)
                n91 = Unbundle By Name(w252) -> ("Data.PID 2 output"=w284:dbl, "Pump On?"=w283:enum16{"Off", "On", "Not Initialized"})
                n92 = Bundle By Name(cluster=w287, "Flow"=w251, "Scale Value"=w285, "Pump On?"=w283, "Cycle Period"=w267, "Density"=w275, "Input Device"=w276, "FL Temp"=w274, "Output"=w266, "Pump's Pressure"=w264, "Pump's Flow"=w265) -> (w262:T10)
                n93 = Bundle By Name(cluster=w286, "Smoothed Array"=w250, "Flow"=w251, "Manual"=w284) -> (w259:T9)
                n94 = call "Update if Clear.vi"("error in (no error)"=w261, "Message Data"=w262, "Queue in"=w263) -> ("error out"=w258:errorcluster)  [unwired: 8 in]
                n95 = Unbundle By Name(w268) -> ("Input Error"=w282:bool, "Output Error"=w278:bool)
                n96 = Unbundle By Name(w252) -> ("Log Started"=w273:bool)
                n97 = call "Update if Clear.vi"("error in (no error)"=w258, "Message Data"=w259, "Queue in"=w260) -> ("error out"=w257:errorcluster)  [unwired: 8 in]
                n98 = case shown="True" w273 {
                  tunnel: [w303 w308] -> w301
                  tunnel: w292 -> [_ w307]
                  tunnel: w252 -> [w302 w306]
                  tunnel: w257 -> [w303 w305]
                  tunnel: [w302 w304] -> w280
                  frame False {
                  }
                  frame True {
                    n99 = call "Write Tags.vi"("error in (no error)"=w305, "State in"=w306) -> ("error out"=w309:errorcluster, "State out"=w310:T13)  [unwired: 8 in]
                    n100 = call "Graph.vi"("error in (no error)"=w309, "notifier out"=w307, "State in"=w310) -> ("error out"=w308:errorcluster, "State out"=w304:T13)  [unwired: 7 in]
                  }
                }
                n101 = Unbundle By Name(w280) -> ("Input Error"=w281:bool, "Output Error"=w277:bool)
                n102 = case shown="False" w278 {
                  tunnel: w277 -> [w312 _]
                  tunnel: w279 -> [w311 _]
                  frame False {
                    n103 = case shown="True" w312 {
                      tunnel: w311 -> [_ w314]
                      frame False {
                      }
                      frame True {
                        # "Pause if there is a new error"
                        n104 = call-poly "Enqueue Message.vi"("Message"="In Error", "Message Queue"=w314) -> ()  [unwired: 8 in, 2 out]
                      }
                    }
                  }
                  frame True {
                  }
                }
                n105 = case shown="False" w282 {
                  tunnel: w281 -> [w316 _]
                  tunnel: w279 -> [w315 _]
                  frame False {
                    n106 = case shown="True" w316 {
                      tunnel: w315 -> [_ w318]
                      frame False {
                      }
                      frame True {
                        # "Pause if there is a new error"
                        n107 = call-poly "Enqueue Message.vi"("Message"="In Error", "Message Queue"=w318) -> ()  [unwired: 8 in, 2 out]
                      }
                    }
                  }
                  frame True {
                  }
                }
                n108 = Bundle By Name(cluster=w280, "First Iteration"=FALSE) -> (w294:T13)
              }
              frame "Idle", Default {
                n109 = Unbundle By Name(w339) -> ("Configuration.Cycle Period"=w338:dbl)
                n110 = call "Update if Clear.vi"("error in (no error)"=w335, "Message Data"=w336, "Queue in"=w337) -> ("error out"=w332:errorcluster)  [unwired: 8 in]
                n111 = call "Update if Clear.vi"("error in (no error)"=w332, "Message Data"=w333, "Queue in"=w334) -> ("error out"=w331:errorcluster)  [unwired: 8 in]
              }
              frame "Paused" {
                # "PID is 0 when paused"
                # "Send\ngraph data"
                # "Enqueue\nlog data"
                n112 = call "Timed Loop Time.vi"("error in (no error)"=w366, "ET since start (s)"=w383, "State in"=w367) -> ("error out"=w385:errorcluster, "State out"=w386:T13)  [unwired: 7 in]
                n113 = call "Inputs.vi"("error in (no error)"=w385, "State in"=w386) -> ("error out"=w370:errorcluster, "State out"=w369:T13)  [unwired: 8 in]
                n114 = Bundle By Name(cluster=w369, "Data.PID 2 output"=0.0) -> (w359:T13)
                n115 = call "Outputs.vi"("error in (no error)"=w370, "State in"=w359) -> ("error out"=w364:errorcluster, "State out"=w365:T13)  [unwired: 8 in]
                n116 = call "Pump Status.vi"("error in (no error)"=w364, "State in"=w365) -> ("error out"=w363:errorcluster, "State out"=w356:T13)  [unwired: 8 in]
                n117 = Unbundle By Name(w356) -> ("Log Started"=w355:bool)
                n118 = case shown="True" w355 {
                  tunnel: w384 -> [_ w393]
                  tunnel: [w387 w392] -> w348
                  tunnel: w356 -> [w388 w391]
                  tunnel: w363 -> [w387 w390]
                  tunnel: [w388 w389] -> w362
                  frame False {
                  }
                  frame True {
                    n119 = call "Write Tags.vi"("error in (no error)"=w390, "State in"=w391) -> ("error out"=w395:errorcluster, "State out"=w394:T13)  [unwired: 8 in]
                    n120 = call "Graph.vi"("error in (no error)"=w395, "notifier out"=w393, "State in"=w394) -> ("error out"=w392:errorcluster, "State out"=w389:T13)  [unwired: 7 in]
                  }
                }
                n121 = Unbundle By Name(w356) -> ("Pump On?"=w378:enum16{"Off", "On", "Not Initialized"})
                n122 = Bundle By Name(cluster=w362, "First Iteration"=FALSE) -> (w361:T13)
                n123 = Unbundle By Name(w359) -> ("Data.Scale Output (g)"=w380:dbl, "Configuration.PID 2 Parameters.Input Device"=w354:T11, "Configuration.Cycle Period"=w353:dbl, "Data.PID 2 output"=w379:dbl, "Data.Pump Flow"=w352:dbl, "Data.Pump Pressure"=w351:dbl)
                n124 = case shown="\"Bronkhorst M13\", \"Bronkhorst M14\"" w354 {
                  tunnel: w359 -> [_ w402 w406]
                  tunnel: [0.0 ("Scale Rate of Change (g/min)") w401 w405] -> w341
                  tunnel: [0.0 ("Density") w400 nan ("Density")] -> w358
                  tunnel: [0.0 ("Density") w399 nan ("Density")] -> w357
                  frame "Default", Default {
                  }
                  frame "Bronkhorst M13", "Bronkhorst M14" {
                    n125 = Unbundle By Name(w402) -> ("Data.Flowmeter Output"=w401:dbl, "Data.Density"=w400:dbl, "Data.FL Temp"=w399:dbl)
                  }
                  frame "Scale Rate of Change" {
                    n126 = Unbundle By Name(w406) -> ("Data.Scale Rate of Change (g/min)"=w405:dbl)
                  }
                }
                n127 = call "Rolling Average.vi"("New Value"=w341, "Old Array"=w343) -> ("Calculated Value"=w340:dbl, "New Array"=w342:dbl[])  [unwired: 8 in]
                n128 = Bundle By Name(cluster=w381, "Flow"=w340, "Scale Value"=w380, "Pump On?"=w378, "Cycle Period"=w353, "Density"=w358, "FL Temp"=w357, "Input Device"=w354, "Pump's Pressure"=w351, "Pump's Flow"=w352) -> (w349:T10)
                n129 = case shown="\"Off\", Default" w378 {
                  tunnel: w379 -> [_ w416]
                  tunnel: [0.0 w416] -> w377
                  frame "Off", Default {
                  }
                  frame "On" {
                  }
                }
                n130 = call "Update if Clear.vi"("error in (no error)"=w348, "Message Data"=w349, "Queue in"=w350) -> ("error out"=w345:errorcluster)  [unwired: 8 in]
                n131 = Unbundle By Name(w361) -> ("Input Error"=w374:bool, "Output Error"=w371:bool)
                n132 = Unbundle By Name(w376) -> ("Input Error"=w375:bool, "Output Error"=w372:bool)
                n133 = Bundle By Name(cluster=w382, "Flow"=w340, "Manual"=w377) -> (w346:T9)
                n134 = case shown="False" w372 {
                  tunnel: w371 -> [w408 _]
                  tunnel: w373 -> [w407 _]
                  frame False {
                    n135 = case shown="True" w408 {
                      tunnel: w407 -> [_ w410]
                      frame False {
                      }
                      frame True {
                        n136 = call-poly "Enqueue Message.vi"("Message"="In Error", "Message Queue"=w410) -> ()  [unwired: 8 in, 2 out]
                      }
                    }
                  }
                  frame True {
                  }
                }
                n137 = case shown="False" w375 {
                  tunnel: w374 -> [w412 _]
                  tunnel: w373 -> [w411 _]
                  frame False {
                    n138 = case shown="True" w412 {
                      tunnel: w411 -> [_ w414]
                      frame False {
                      }
                      frame True {
                        n139 = call-poly "Enqueue Message.vi"("Message"="In Error", "Message Queue"=w414) -> ()  [unwired: 8 in, 2 out]
                      }
                    }
                  }
                  frame True {
                  }
                }
                n140 = call "Update if Clear.vi"("error in (no error)"=w345, "Message Data"=w346, "Queue in"=w347) -> ("error out"=w344:errorcluster)  [unwired: 8 in]
              }
            }
            n141 = Subtract(x=w240, y=w241) -> (x-y=→"Period (s)":dbl)
          }
          frame "Stop" {
            # "Stop - Flush the message queue of any pending \"Log\" messages. Call 'Flush Data to Log File.vi' so any pending data is not lost."
            n142 = Unbundle By Name(w426) -> ("State"=w429:T8)
            n143 = Unbundle By Name(w426) -> ("Configuration.Cycle Period"=w425:dbl)
            n144 = case shown="\"Measuring\", Default" w429 {
              tunnel: [w436 w442] -> w422
              tunnel: w427 -> [w432 w442]
              tunnel: w431 -> [_ _]
              tunnel: w430 -> [w440 _]
              tunnel: w426 -> [w434 w441]
              tunnel: [w438 w441] -> w424
              frame "Measuring", Default {
                # "If the system is logging, stop logging."
                n145 = call "Close.vi"("error in (no error)"=w432, "State in"=w434) -> ("error out"=w433:errorcluster, "State out"=w435:T13)  [unwired: 8 in]
                n146 = Bundle By Name(cluster=w435, "State"=State_Enum."Idle") -> (w438:T13)
                n147 = call-poly "Enqueue Message.vi"("error in (no error)"=w433, "Message"="Logging Stopped", "Message Queue"=w440) -> ("error out"=w436:errorcluster)  [unwired: 7 in, 1 out]
              }
              frame "Idle" {
                # "The system is already idle. Ignore the \"Stop\" message."
              }
            }
            n148 = call "Update if Clear.vi"("error in (no error)"=w422, "Message Data"=w424, "Queue in"=w423) -> ("error out"=w419:errorcluster)  [unwired: 8 in]
            n149 = call "Update if Clear.vi"("error in (no error)"=w419, "Message Data"=w420, "Queue in"=w421) -> ("error out"=w418:errorcluster)  [unwired: 8 in]
          }
          frame "Pause" {
            # "Stop - Flush the message queue of any pending \"Log\" messages. Call 'Flush Data to Log File.vi' so any pending data is not lost."
            n150 = Unbundle By Name(w452) -> ("State"=w458:T8, "First Iteration"=w456:bool)
            n151 = Unbundle By Name(w452) -> ("Configuration.Cycle Period"=w451:dbl)
            n152 = case shown="True" w456 {
              tunnel: w452 -> [w461 w466]
              tunnel: [w461 w467] -> w453
              tunnel: w455 -> [w460 w464]
              tunnel: [w460 w463] -> w454
              frame False {
              }
              frame True {
                # "If we load to a paused state we initialize"
                n153 = call "Initialize.vi"("error in (no error)"=w464, "State in"=w466) -> ("error out"=w463:errorcluster, "Pump Initialized"=w468:bool, "State out"=w465:T13)  [unwired: 7 in]
                n154 = case shown="True" w468 {
                  tunnel: [enum16{"Off", "On", "Not Initialized"}."Not Initialized" ("Pump On?") enum16{"Off", "On", "Not Initialized"}."Off" ("Pump On?")] -> w469
                  tunnel: [_ FALSE] -> w462
                  frame False {
                  }
                  frame True {
                  }
                }
                n155 = Bundle By Name(cluster=w465, "Pump On?"=w469, "First Iteration"=w462) -> (w467:T13)
              }
            }
            n156 = case shown="\"Measuring\", Default" w458 {
              tunnel: [w477 w485 w489] -> w448
              tunnel: w454 -> [w475 w485 w489]
              tunnel: w459 -> [w481 _ _]
              tunnel: w453 -> [w476 w483 w487]
              tunnel: [w479 w482 w486] -> w449
              frame "Measuring", Default {
                # "If the system is logging, stop logging."
                n157 = call "Pause.vi"("error in (no error)"=w475, "State in"=w476) -> ("error out"=w474:errorcluster, "State out"=w473:T13)  [unwired: 8 in]
                n158 = Bundle By Name(cluster=w473, "State"=State_Enum."Paused") -> (w479:T13)
                n159 = call-poly "Enqueue Message.vi"("error in (no error)"=w474, "Message"="Logging Stopped", "Message Queue"=w481) -> ("error out"=w477:errorcluster)  [unwired: 7 in, 1 out]
              }
              frame "Idle" {
                # "The system is already idle. Ignore the \"Stop\" message."
                n160 = Bundle By Name(cluster=w483, "State"=State_Enum."Paused") -> (w482:T13)
              }
              frame "Paused" {
                n161 = Bundle By Name(cluster=w487, "State"=State_Enum."Paused") -> (w486:T13)
              }
            }
            n162 = call "Update if Clear.vi"("error in (no error)"=w448, "Message Data"=w449, "Queue in"=w450) -> ("error out"=w444:errorcluster)  [unwired: 8 in]
            n163 = call "Update if Clear.vi"("error in (no error)"=w444, "Message Data"=w446, "Queue in"=w447) -> ("error out"=w445:errorcluster)  [unwired: 8 in]
          }
          frame "Update Settings" {
            w503 = T14 {"Cycle Period"=0.0, "Ismatech"={"VISA resource name"="", "Simulated?"=FALSE, "Pump Number"=1.0, "Reverse?"=FALSE}, "Masterflex"={"VISA resource name"="", "Simulated?"=FALSE, "Pump Number"=1.0, "Reverse?"=FALSE}, "Mettler"={"VISA resource name"="", "Simulated?"=FALSE}, "Bronkhorst M13 Flow Meter"={"VISA resource name"="", "Simulated?"=FALSE, "Smoothing Steps"=1}, "PID 2 Parameters"={"Input Device"=enum."Bronkhorst M13", "Output Device"=enum."Ismatec ISM 831C", "Setpoint"=0.0, "PID gains"={"proportional gain (Kc)"=1.0, "integral time (Ti, min)"=0.01, "derivative time (Td, min)"=0.0}}, "Manual Entry"=0.0, "Auto?"=TRUE, "output range"={"output high"=100.0, "output low"=0.0}, "Tacmina Settings"={"Analog DAQ Task"="", "Digital DAQ Task"=""}, "KNF SIMDOS Settings"={"VISA resource name"="", "Simulated?"=TRUE}, "ASIA Pump C"={"ASIA Pump #"=0, "channel"=0, "Simulated"=FALSE}, "VICI Settings"={"VISA resource name"="", "Simulated?"=FALSE, "Pump Letter"="", "Reverse?"=FALSE}, "FLOM Settings"={"VISA resource name"="", "Simulated?"=TRUE, "Pump Number"=0.0}, "SSI PR/LD Settings"={"VISA resource name"="", "Simulated?"=FALSE}, "Masterflex 75211 Settings"={"Analog DAQ Task"="", "Digital DAQ Task"=""}, "SSI P40 Settings"={"VISA resource name"="", "Simulated?"=TRUE}, "Ismatech 3 Channel Settings"={"VISA resource name"="", "Pump Number"=1, "Channel Number"=0, "Simulated?"=TRUE, "Reverse?"=FALSE}, "Bronkhorst M14 Settings"={"VISA resource name"="", "Simulated?"=FALSE, "Smoothing Steps"=1}}  # Configuration
            # "New settings are available, update the current ones stored in the shift register with the settings sent as part of the message"
            n164 = Variant To Data(error in=w504, type=w503, Variant=w505) -> (data=w499:T14, error out=w498:errorcluster)
            n165 = Bundle By Name(cluster=w500, "Configuration"=w499) -> (w496:T13)
            n166 = Unbundle By Name(w496) -> ("Configuration.Cycle Period"=w497:dbl)
            n167 = Unbundle By Name(w496) -> ("Configuration.PID 2 Parameters.Input Device"=w493:T11, "Configuration.Bronkhorst M13 Flow Meter.Smoothing Steps"=w492:i32, "Configuration.Bronkhorst M14 Settings.Smoothing Steps"=w491:i32)
            n168 = case shown="\"Bronkhorst M13\"" w493 {
              tunnel: w492 -> [_ w507 _]
              tunnel: w491 -> [_ _ w508]
              tunnel: [1 ("Smoothing Steps") w507 w508] -> w495
              frame Default {
              }
              frame "Bronkhorst M13" {
              }
              frame "Bronkhorst M14" {
              }
            }
            n169 = Initialize Array(0.0 ("element"), w495) -> (w490:dbl[])
          }
          frame "Exit" {
            # "Release the Logging queue reference"
            # "Don't check the error out. The UI message queue may have already been released."
            # "Stop the VI"
            # "Exit - Send the Exit message to the UI Message Handler.  Call 'Flush Data to Log File.vi' so any pending data is not lost."
            n170 = Release Queue(queue=w516, error in (no error)=w519) -> (error out=w515:errorcluster)  [unwired: 1 in, 2 out]
            n171 = call-poly "Enqueue Message.vi"("Priority Message? (F)"=TRUE, "Message"="Exit", "Message Queue"=w520) -> ("error out"=w514:errorcluster)  [unwired: 7 in, 1 out]
            n172 = call <vilib>:"Clear Errors.vi"("error in (no error)"=w514) -> ()  [unwired: 5 in, 2 out]
            n173 = Unbundle By Name(w511) -> ("Configuration.Cycle Period"=w510:dbl)
            n174 = Merge Errors(w515) -> (w521:errorcluster)
          }
          frame "---Copy This Frame---" {
            # "Duplicate this frame when creating new messages.  Change this comment in the duplicated frame to describe this message."
            n175 = Merge Errors(w529) -> (w528:errorcluster)
            n176 = Unbundle By Name(w525) -> ("Configuration.Cycle Period"=w524:dbl)
          }
          frame "In Error" {
            # "Duplicate this frame when creating new messages.  Change this comment in the duplicated frame to describe this message."
            n177 = Unbundle By Name(w558) -> ("Configuration.Cycle Period"=w557:dbl)
            n178 = Merge Errors(w563) -> (w561:errorcluster)
            n179 = call "Initialize.vi"("error in (no error)"=w561, "State in"=w558) -> ("error out"=w535:errorcluster, "Pump Initialized"=w562:bool, "State out"=w549:T13)  [unwired: 7 in]
            n180 = Unbundle By Name(w549) -> ("Configuration.Cycle Period"=w548:dbl, "Pump On?"=w546:enum16{"Off", "On", "Not Initialized"}, "Configuration.PID 2 Parameters.Input Device"=w544:T11, "Configuration.PID 2 Parameters.Output Device"=w547:T12, "Current Setpoint"=w545:dbl)
            n181 = Unbundle By Name(w549) -> ("Data"=w554:T31)
            n182 = Unbundle By Name(w554) -> ("Flowmeter Output"=w531:dbl, "Density"=w553:dbl, "FL Temp"=w552:dbl, "Scale Rate of Change (g/min)"=w543:dbl, "Pump Flow"=w550:dbl, "Pump Pressure"=w551:dbl)
            n183 = call "Rolling Average.vi"("New Value"=w531, "Old Array"=w533) -> ("Calculated Value"=w530:dbl, "New Array"=w532:dbl[])  [unwired: 8 in]
            n184 = Bundle By Name(cluster=w556, "Flow"=w530, "Density"=w553, "FL Temp"=w552, "Scale Value"=w543, "Pump On?"=w546, "Cycle Period"=w548, "Input Device"=w544, "Output"=w547, "Pump's Pressure"=w551, "Pump's Flow"=w550) -> (w538:T10)
            n185 = case shown="\"Bronkhorst M13\", \"Bronkhorst M14\"" w544 {
              tunnel: w530 -> [_ w565 _]
              tunnel: w543 -> [_ _ w566]
              tunnel: [0.0 ("Scale Rate of Change (g/min)") w565 w566] -> w542
              frame "Default", Default {
              }
              frame "Bronkhorst M13", "Bronkhorst M14" {
              }
              frame "Scale Rate of Change" {
              }
            }
            n186 = Bundle By Name(cluster=w555, "Flow"=w542, "Manual"=w545, "Pump Status"=w546) -> (w537:T9)
            n187 = call "Update if Clear.vi"("error in (no error)"=w535, "Message Data"=w538, "Queue in"=w539) -> ("error out"=w536:errorcluster)  [unwired: 8 in]
            n188 = call "Update if Clear.vi"("error in (no error)"=w536, "Message Data"=w537, "Queue in"=w540) -> ("error out"=w534:errorcluster)  [unwired: 8 in]
            n189 = case shown="True" w562 {
              tunnel: w541 -> [w571 w575]
              tunnel: w534 -> [w570 w574]
              tunnel: [w568 w577] -> w560
              tunnel: w549 -> [w568 w577]
              tunnel: [w567 w573] -> w559
              frame False {
                n190 = Wait (ms)(milliseconds to wait=u32 5000) -> ()  [unwired: 1 out]
                n191 = call-poly "Enqueue Message.vi"("error in (no error)"=w570, "Message"="In Error", "Message Queue"=w571) -> ("error out"=w567:errorcluster)  [unwired: 7 in, 1 out]
              }
              frame True {
                n192 = call-poly "Enqueue Message.vi"("error in (no error)"=w574, "Message"="Measure", "Message Queue"=w575) -> ("error out"=w573:errorcluster)  [unwired: 7 in, 1 out]
              }
            }
          }
          frame Default {
            # "'Default' case only runs if there is a message that isn't defined in any of the other cases.  Output a programming error."
            n193 = Unbundle By Name(w586) -> ("Configuration.Cycle Period"=w585:dbl)
            n194 = Concatenate Strings("The invalid message string " ("string"), w579, " was received in the Feed Module Engine." ("string")) -> (w581:string)
            n195 = Bundle By Name(cluster=errorcluster {"status"=TRUE, "code"=1, "source"=""} ("error constant"), "source"=w581) -> (w580:errorcluster)
          }
        }
        n196 = Unbundle By Name(w41) -> ("State"=w40:T8, "Configuration.Cycle Period"=w38:dbl)
        n197 = call "Error Handler.vi"("error in (no error)"=w47, "Message Queue"=w45) -> ("dup error in"=w46:errorcluster)  [unwired: 8 in, 1 out]
        n198 = case shown="\"Paused\"" w40 {
          tunnel: [w53 1 1] -> w39
          tunnel: w38 -> [w53 _ _]
          frame "Measuring" {
          }
          frame "Idle" {
          }
          frame "Paused" {
          }
        }
        n199 = node-c288(w39) -> ()  [unwired: 1 in, 1 out]
      }
      n200 = feedback-in #1(w8) -> ()
      n201 = node-c288(w17) -> ()  [unwired: 1 out]
    }
    frame Error {
    }
  }
  "error out" <- w3
